vi "BasicVariantAttr.vi"() -> ()   [LabVIEW 2010]
panel:
  out "Everybody":T1(array[cluster])
  out "Person of interest":T2
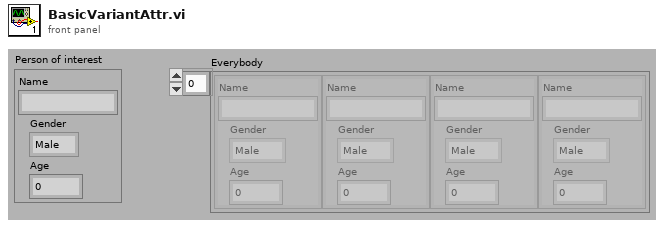
[diagram p1: front panel]
types:
  T1 = cluster{"Name":string, "Gender":enum16{"Male", "Female"}, "Age":dbl}[]
  T2 = cluster{"Name":string, "Gender":enum16{"Male", "Female"}, "Age":dbl}
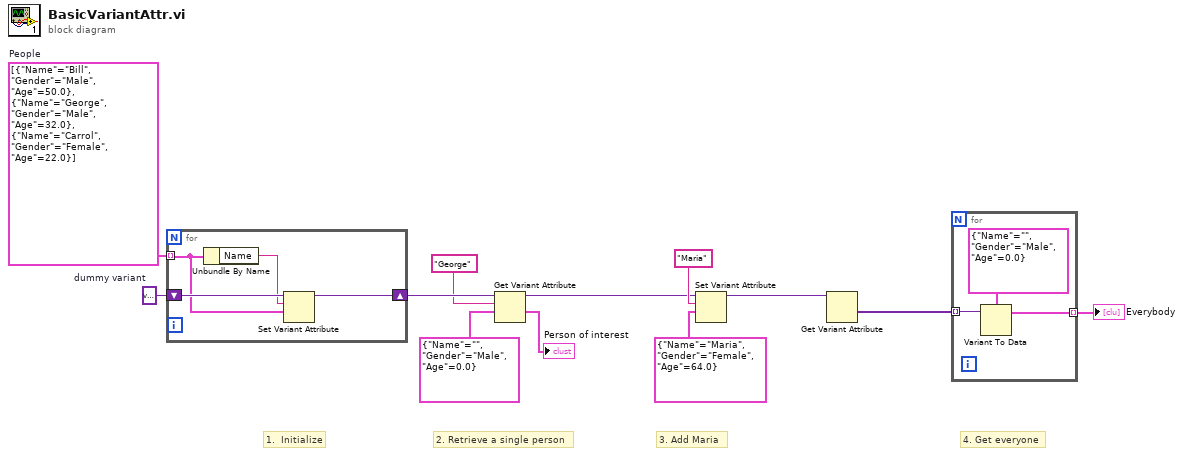
[diagram p0: block diagram]
diagram:
  w12 = T1 [{"Name"="Bill", "Gender"=enum."Male", "Age"=50.0}, {"Name"="George", "Gender"=enum."Male", "Age"=32.0}, {"Name"="Carrol", "Gender"=enum."Female", "Age"=22.0}]  # People
  w11 = variant  # dummy variant
  # "4. Get everyone"
  # "3. Add Maria"
  # "2. Retrieve a single person"
  # "1.  Initialize"
  n1 = for {
    tunnel: w12 -> [w14] mode=indexing
    shift-right: [w13] -> w10
    shift-left: w11 -> [w16]
    n2 = Unbundle By Name(w14) -> ("Name"=w15:string)
    n3 = Set Variant Attribute(Variant=w16, name=w15, value=w14) -> (Variant out=w13:variant)  [unwired: 1 in, 2 out]
  }
  n4 = Get Variant Attribute(Variant=w10, name="George", default value (empty Variant)=T2 {"Name"="", "Gender"=enum."Male", "Age"=0.0} ("Person")) -> (duplicate Variant=w4:variant, value=→"Person of interest":T2)  [unwired: 1 in, 2 out]
  n5 = Set Variant Attribute(Variant=w4, name="Maria", value=T2 {"Name"="Maria", "Gender"=enum."Female", "Age"=64.0} ("Person")) -> (Variant out=w3:variant)  [unwired: 1 in, 2 out]
  n6 = Get Variant Attribute(Variant=w3) -> (values=w2:variant[])  [unwired: 3 in, 3 out]
  n7 = for {
    tunnel: w2 -> [w19] mode=indexing
    tunnel: [w18] -> w1 mode=indexing
    n8 = Variant To Data(Variant=w19, type=T2 {"Name"="", "Gender"=enum."Male", "Age"=0.0} ("Person")) -> (data=w18:T2)  [unwired: 1 in, 1 out]
  }
  "Everybody" <- w1
